vi "CheckVariantAttributes.vi"(8 "error in (no error)":errorcluster, 11 "Variant In":variant) -> (0 "error out":errorcluster, 3 "Variant Out":variant)   [LabVIEW 2020]
uses:
  typedefs/Schedule Types/Schedule--Constant.ctl
  typedefs/Schedule Types/Schedule--Ramp.ctl
  typedefs/Signal Type - enum.ctl
  typedefs/Schedule Types/Schedule--Function Generator.ctl
  typedefs/Schedule Types/Schedule--Formula.ctl
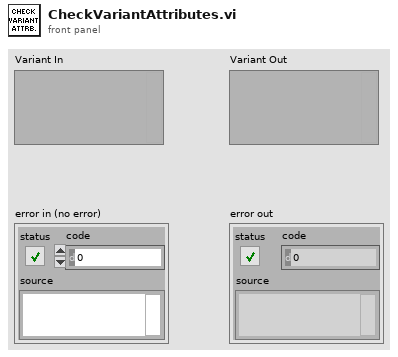
[diagram p1: front panel]
types:
  T1 = typedef "Schedule--Formula.ctl" = cluster{"formula":string, "formula length (nm)":dbl, "formula resolution (nm)":dbl}
  T2 = typedef "Schedule--Function Generator.ctl" = cluster{"Min Value":dbl, "Max Value":dbl, "Duty Cycle (%)":dbl, "Signal Type":T3, "Cycle Number":dbl, "Phase (degrees)":dbl}
  T3 = typedef "Signal Type - enum.ctl" = enum16{"Sine Wave", "Triangle Wave", "Square Wave", "Sawtooth Wave"}
  T4 = typedef "Schedule--Ramp.ctl" = cluster{"Start":dbl, "End":dbl}
  T5 = typedef "Schedule--Constant.ctl" = cluster{"Value":dbl}
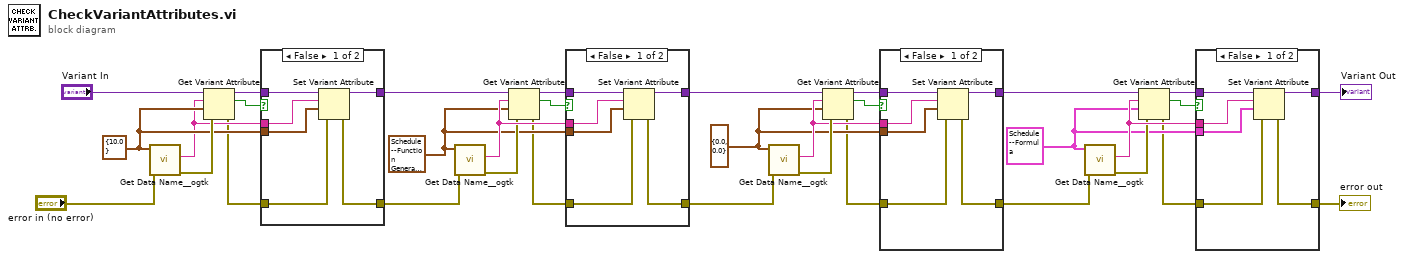
[diagram p0: block diagram]
diagram:
  w11 = T1 {"formula"="1*(step(170-t)*cos(0.62831853071*t)+step(t-170)*cos(0.62831853071*(t-170))*(-1))", "formula length (nm)"=340.0, "formula resolution (nm)"=0.001} ("Formula")
  w23 = T2 {"Min Value"=0.0, "Max Value"=0.0, "Duty Cycle (%)"=0.0, "Signal Type"=enum."Square Wave", "Cycle Number"=0.0, "Phase (degrees)"=0.0} ("Fn. Gen")
  w17 = T4 {"Start"=0.0, "End"=0.0} ("Ramp")
  w30 = T5 {"Value"=10.0} ("Constant")
  n1 = call <userlib>:"Get Data Name__ogtk.vi"("error in (no error)"="error in (no error)", "Data"=w30) -> ("error out"=w33:errorcluster, "Data Name"=w29:string)  [unwired: 7 in, 1 out]
  n2 = Get Variant Attribute(Variant="Variant In", name=w29, default value (empty Variant)=w30, error in=w33) -> (duplicate Variant=w31:variant, found=w32:bool, error out=w8:errorcluster)  [unwired: 1 out]
  n3 = case shown="False" w32 {
    tunnel: w31 -> [w40 w42]
    tunnel: w30 -> [w38 _]
    tunnel: w29 -> [w39 _]
    tunnel: [w37 w42] -> w24
    tunnel: w8 -> [w35 w41]
    tunnel: [w36 w41] -> w6
    frame False {
      n4 = Set Variant Attribute(Variant=w40, name=w39, value=w38, error in=w35) -> (Variant out=w37:variant, error out=w36:errorcluster)  [unwired: 1 out]
    }
    frame True {
    }
  }
  n5 = call <userlib>:"Get Data Name__ogtk.vi"("error in (no error)"=w6, "Data"=w23) -> ("error out"=w25:errorcluster, "Data Name"=w28:string)  [unwired: 7 in, 1 out]
  n6 = Get Variant Attribute(Variant=w24, name=w28, default value (empty Variant)=w23, error in=w25) -> (duplicate Variant=w27:variant, found=w26:bool, error out=w7:errorcluster)  [unwired: 1 out]
  n7 = case shown="False" w26 {
    tunnel: w27 -> [w48 w50]
    tunnel: w23 -> [w46 _]
    tunnel: w28 -> [w47 _]
    tunnel: [w45 w50] -> w18
    tunnel: [w43 w49] -> w4
    tunnel: w7 -> [w44 w49]
    frame False {
      n8 = Set Variant Attribute(Variant=w48, name=w47, value=w46, error in=w44) -> (Variant out=w45:variant, error out=w43:errorcluster)  [unwired: 1 out]
    }
    frame True {
    }
  }
  n9 = call <userlib>:"Get Data Name__ogtk.vi"("error in (no error)"=w4, "Data"=w17) -> ("error out"=w22:errorcluster, "Data Name"=w19:string)  [unwired: 7 in, 1 out]
  n10 = Get Variant Attribute(Variant=w18, name=w19, default value (empty Variant)=w17, error in=w22) -> (duplicate Variant=w20:variant, found=w21:bool, error out=w5:errorcluster)  [unwired: 1 out]
  n11 = case shown="False" w21 {
    tunnel: w20 -> [w56 w58]
    tunnel: w17 -> [w54 _]
    tunnel: w19 -> [w55 _]
    tunnel: [w53 w58] -> w12
    tunnel: [w52 w57] -> w3
    tunnel: w5 -> [w51 w57]
    frame False {
      n12 = Set Variant Attribute(Variant=w56, name=w55, value=w54, error in=w51) -> (Variant out=w53:variant, error out=w52:errorcluster)  [unwired: 1 out]
    }
    frame True {
    }
  }
  n13 = call <userlib>:"Get Data Name__ogtk.vi"("error in (no error)"=w3, "Data"=w11) -> ("error out"=w13:errorcluster, "Data Name"=w16:string)  [unwired: 7 in, 1 out]
  n14 = Get Variant Attribute(Variant=w12, name=w16, default value (empty Variant)=w11, error in=w13) -> (duplicate Variant=w15:variant, found=w14:bool, error out=w2:errorcluster)  [unwired: 1 out]
  n15 = case shown="False" w14 {
    tunnel: w15 -> [w64 w66]
    tunnel: w11 -> [w62 _]
    tunnel: w16 -> [w63 _]
    tunnel: [w61 w66] -> w10
    tunnel: w2 -> [w60 w65]
    tunnel: [w59 w65] -> w1
    frame False {
      n16 = Set Variant Attribute(Variant=w64, name=w63, value=w62, error in=w60) -> (Variant out=w61:variant, error out=w59:errorcluster)  [unwired: 1 out]
    }
    frame True {
    }
  }
  "Variant Out" <- w10
  "error out" <- w1
